vi "Write YState.vi"(7 "OPC UA AI list":string[](array[string]), 8 "error in (no error)":errorcluster, 10 "Y_State":T1 {"Y" format="%.2f"; "Y_preSet" format="%.2f"; "SP" step=0.01 format="%.2f"; "Y_Set" format="%.2f"; "PV" step=0.01 format="%.2f"; "SP_Set" step=0.01 format="%.2f"}, 11 "OPC UA server refnum in":T6) -> (0 "error out":errorcluster, 3 "OPC UA server refnum out":T6)   [LabVIEW 2019, in "OPC addons.lvlib"]
uses:
  OPC addons.lvlib
  <vilib>/OPCUA/controls/OPC UA Server Refnum.ctl
  Reg/ctl/Ys.ctl
  Reg/ctl/Y.ctl
  Reg/ctl/Y_source.ctl
  Reg/ctl/Y_state.ctl
  Inputs/Ctl/Parameter State short.ctl
  Reg/ctl/Y_short.ctl
  <vilib>/OPCUA/controls/Write Status.ctl
  <vilib>/OPCUA/server/Write Variant.vi
  Inputs/Inputs.lvlib
  Reg/control.lvlib
  <vilib>/OPCUA/NI OPC UA Server.lvlib
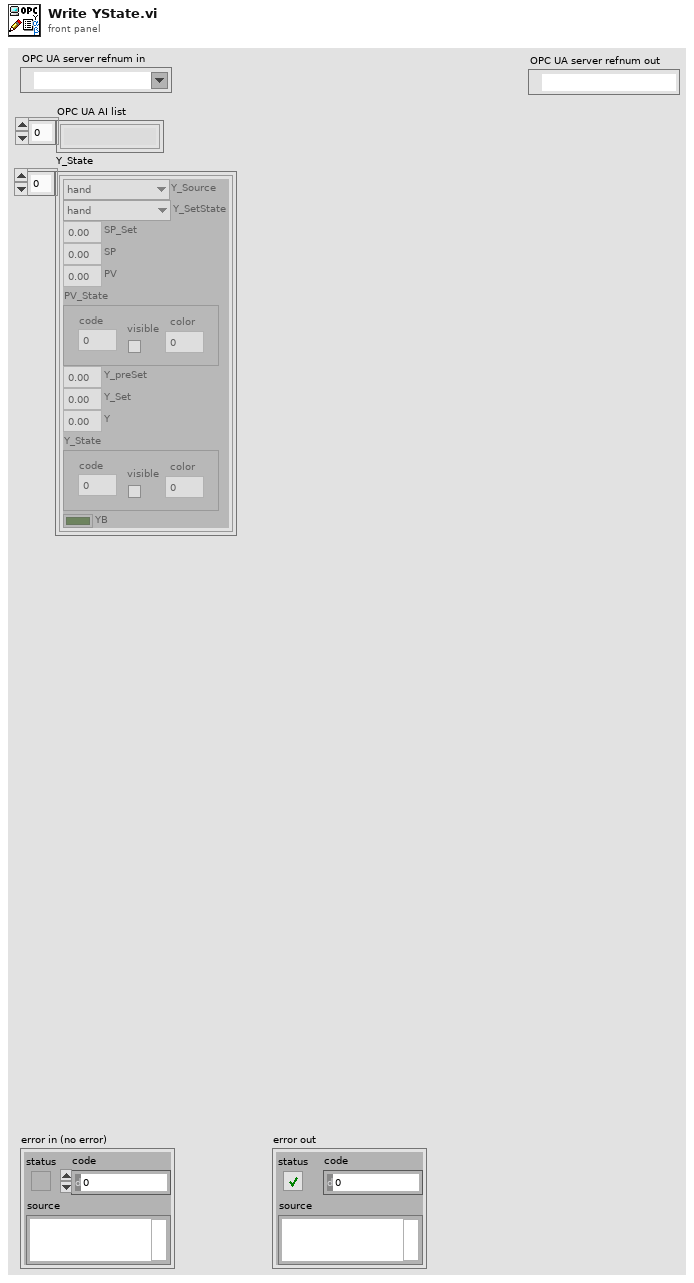
[diagram p1: front panel]
types:
  T1 = typedef "control.lvlib/Ys.ctl" = T2[]
  T2 = typedef "control.lvlib/Y.ctl" = cluster{"Y_Source":T3, "Y_SetState":T4, "SP_Set":dbl, "SP":dbl, "PV":dbl, "PV_State":T5, "Y_preSet":dbl, "Y_Set":dbl, "Y":dbl, "Y_State":T5, "YB":bool}
  T3 = typedef "control.lvlib/Y_source.ctl" = enum8{"initialize", "local disabled", "local hand", "hand", "auto", "dist"}
  T4 = typedef "control.lvlib/Y_state.ctl" = enum8{"initialize", "alarm", "min", "stop", "hand", "auto", "max"}
  T5 = typedef "Inputs.lvlib/Parameter State short.ctl" = cluster{"code":i32, "visible":bool, "color":u32}
  T6 = typedef "OPC UA Server Refnum.ctl" = refnum<k21>
  T7 = typedef "control.lvlib/Y_short.ctl" = cluster{"Y_Source":u8, "Y_SetState":u8, "SP_Set":dbl, "SP":dbl, "PV":dbl, "PV_State":T5, "Y_preSet":dbl, "Y_Set":dbl, "Y":dbl, "Y_State":T5, "YB":bool}
  T8 = typedef "Write Status.ctl" = u32
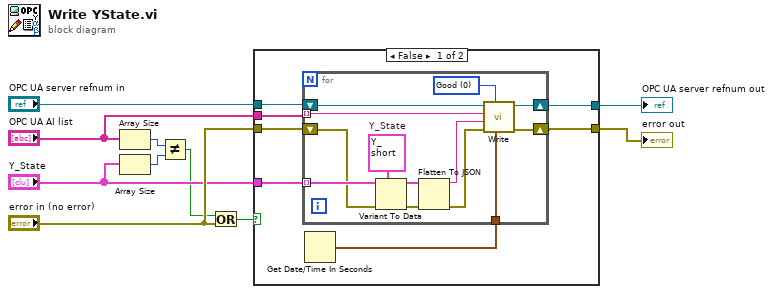
[diagram p0: block diagram]
diagram:
  n1 = Array Size(array="OPC UA AI list") -> (size(s)=w3:i32)
  n2 = Array Size(array="Y_State") -> (size(s)=w2:i32)
  n3 = Not Equal?(x=w3, y=w2) -> (x != y?=w1:bool)
  n4 = Or(x=w1, y="error in (no error)") -> (x .or. y?=w6:bool)
  n5 = case shown="False" w6 {
    tunnel: "OPC UA server refnum in" -> [w14 w32]
    tunnel: [w16 w32] -> w9
    tunnel: [w15 w31] -> w8
    tunnel: "OPC UA AI list" -> [w13 _]
    tunnel: "error in (no error)" -> [w12 w31]
    tunnel: "Y_State" -> [w11 _]
    frame False {
      n6 = Get Date/Time In Seconds() -> (seconds since 1Jan1904=w17:timestamp)
      n7 = for {
        tunnel: w17 -> [w29]
        tunnel: w13 -> [w28] mode=indexing
        shift-right: [w26] -> w16
        shift-left: w14 -> [w30]
        shift-right: [w25] -> w15
        shift-left: w12 -> [w18]
        tunnel: w11 -> [w21] mode=indexing
        w22 = T7 {"Y_Source"=3, "Y_SetState"=3, "SP_Set"=0.0, "SP"=0.0, "PV"=0.0, "PV_State"={"code"=0, "visible"=FALSE, "color"=0}, "Y_preSet"=0.0, "Y_Set"=0.0, "Y"=0.0, "Y_State"={"code"=0, "visible"=FALSE, "color"=0}, "YB"=FALSE}  # Y_State
        w24 = T8 0 items=["Good"=0, "Uncertain"=1073741824, "Uncertain_InitialValue"=1083310080, "Uncertain_LastUsableValue"=1083179008, "Uncertain_SensorNotAccurate"=1083375616, "Uncertain_EngineeringUnitsExceeded"=1083441152, "Bad"=2147483648, "Bad_NoCommunication"=2150694912, "Bad_NotReadable"=2151284736, "Bad_NotWritable"=2151350272, "Bad_OutOfRange"=2151415808, "Bad_WaitingForInitialData"=2150760448] ("node status")
        n8 = Variant To Data(error in=w18, type=w22, Variant=w21) -> (data=w20:T7, error out=w19:errorcluster)
        n9 = Flatten To JSON(anything=w20, error in (no error)=w19) -> (JSON string=w27:string, 11:w23:errorcluster)  [unwired: 1 in]
        n10 = call-poly <vilib>:"Write.vi"("timestamp (current time)"=w29, "node status"=w24, "error in (no error)"=w23, "value"=w27, "node ID"=w28, "OPC UA server refnum in"=w30) -> ("error out"=w25:errorcluster, "OPC UA server refnum out"=w26:T6)  [unwired: 3 in, 1 out]
      }
    }
    frame True {
    }
  }
  "OPC UA server refnum out" <- w9
  "error out" <- w8
